vi "Add Element.vi"(8 "element":string, 9 "category":string, 10 "Value":variant, 11 "Datastore.Dictionaries in":refnum<class "Datastore.Dictionaries.lvclass">) -> (0 "element out":string, 1 "category out":string, 3 "Datastore.Dictionaries":refnum<class "Datastore.Dictionaries.lvclass">)   [LabVIEW 2021, in "Bananas.lvlib" / "Datastore.Dictionaries.lvclass"]
uses:
  Datastore.Dictionaries.lvclass
  Datastore.Dictionaries.lvclass/Datastore.Dictionaries.ctl
  <vilib>/LabVIEW Open Source Project/Data Manipulation/TypeDescriptor/TypeDescriptor_GetName.vi
  <vilib>/LabVIEW Open Source Project/Data Manipulation/TypeDescriptor/TypeDescriptor_GetPString.vi
  <vilib>/LabVIEW Open Source Project/Data Manipulation/Variant/OpenVariant.lvlib
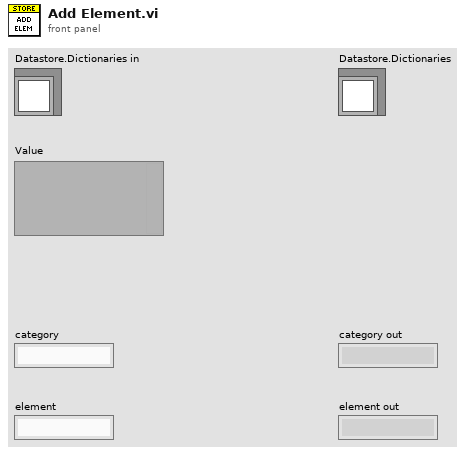
[diagram p1: front panel]
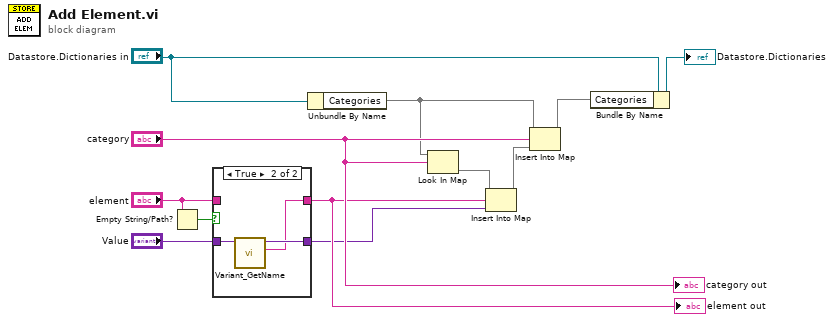
[diagram p0: block diagram]
diagram:
  n1 = Empty String/Path?(string/path="element") -> (empty?=w5:bool)
  n2 = case shown="True" w5 {
    tunnel: "element" -> [w14 _]
    tunnel: [w14 w15] -> w3
    tunnel: "Value" -> [w13 w17]
    tunnel: [w13 w16] -> w1
    frame False {
    }
    frame True {
      n3 = call <vilib>:"Variant_GetName.vi"("Variant"=w17) -> ("Name"=w15:string, "Variant dup"=w16:variant)  [unwired: 8 in, 1 out]
    }
  }
  "element out" <- w3
  n4 = Unbundle By Name("Datastore.Dictionaries in") -> ("Categories"=w11:map{string, map{string, variant}})
  n5 = Look In Map(map=w11, key="category") -> (value=w6:map{string, variant})  [unwired: 1 in, 1 out]
  n6 = Insert Into Map(map in=w6, key=w3, value=w1) -> (map out=w8:map{string, variant})  [unwired: 2 out]
  n7 = Insert Into Map(map in=w11, key="category", value=w8) -> (map out=w7:map{string, map{string, variant}})  [unwired: 2 out]
  n8 = Bundle By Name(cluster="Datastore.Dictionaries in", "Categories"=w7) -> (→"Datastore.Dictionaries":refnum<class "Datastore.Dictionaries.lvclass">)
  "category out" <- "category"
